vi "Measurement Logic.vi"() -> ()   [LabVIEW 2020, in "IVI Scope Measurement.lvlib"]
uses:
  IVI Scope Measurement.lvlib
  Measurement Configuration.ctl
  Measurement Results.ctl
  <vilib>/MeasurementLink/MeasurementLink Measurement Server/Measure Call Context/Measure Call Context.lvclass
  <vilib>/MeasurementLink/MeasurementLink Measurement Server/Measure Call Context/Reserve Sessions - 1Pin.vi
  IVI Scope Instrument/IVI Scope Instrument.lvlib
  <vilib>/MeasurementLink/MeasurementLink Session Management V1/Session Reservation/Session Reservation.lvclass
panel:
  out "measure call context out":refnum<class "Measure Call Context.lvclass">
  in  "measure call context in":refnum<class "Measure Call Context.lvclass">
  out "measurement results":T1
  in  "measurement configuration":T2={"Pin Name"="", "Time Per Record"=0.0, "Minimum Record Length"=0, "Trigger Level"=0.0, "Vertical Range"=0.0, "Vertical Offset"=10.0, "Probe Attenuation"=1.0, "Vertical Coupling"=1} {"Vertical Coupling" items=["AC", "DC", "GND"]}
  out "error out":errorcluster
  in  "error in":errorcluster
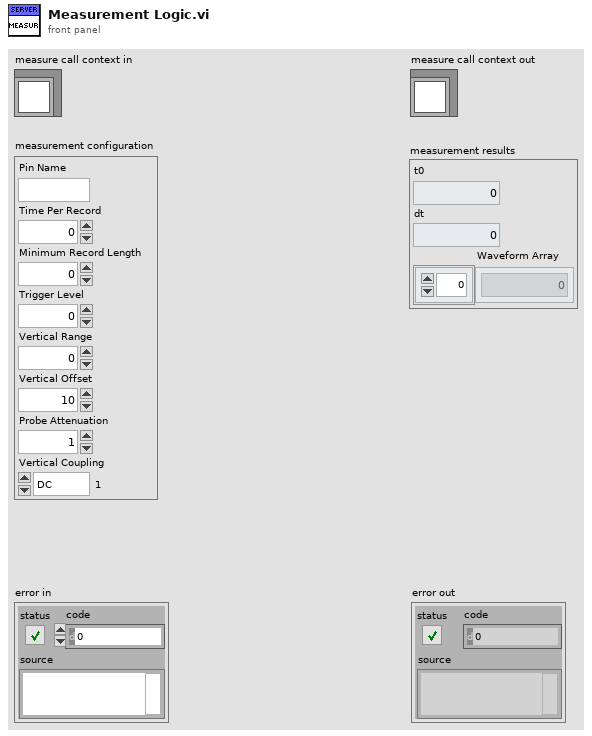
[diagram p1: front panel]
types:
  T1 = typedef "IVI Scope Measurement.lvlib/Measurement Results.ctl" = cluster{"t0":dbl, "dt":dbl, "Waveform Array":dbl[]}
  T2 = typedef "IVI Scope Measurement.lvlib/Measurement Configuration.ctl" = cluster{"Pin Name":string, "Time Per Record":dbl, "Minimum Record Length":i32, "Trigger Level":dbl, "Vertical Range":dbl, "Vertical Offset":dbl, "Probe Attenuation":dbl, "Vertical Coupling":u32}
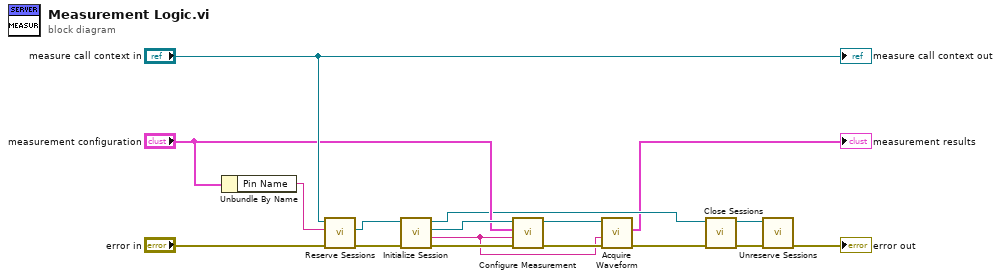
[diagram p0: block diagram]
diagram:
  n1 = Unbundle By Name("measurement configuration") -> ("Pin Name"=w16:string)
  n2 = call-poly <vilib>:"Reserve Sessions.vi"("error in"="error in", "pin or relay name"=w16, "measurement context in"="measure call context in") -> ("error out"=w13:errorcluster, "session reservation out"=w15:refnum<class "Session Reservation.lvclass">)  [unwired: 6 in, 1 out]
  n3 = call "Initialize Session.vi"("error in"=w13, "session reservation in"=w15) -> ("error out"=w12:errorcluster, "channel list"=w1:string, "session"=w11:refnum<k15>, "session reservation out"=w5:refnum<class "Session Reservation.lvclass">)  [unwired: 6 in]
  n4 = call "Configure Measurement.vi"("error in (no error)"=w12, "Channel Name"=w1, "measurement configuration"="measurement configuration", "IVI Refnum in"=w11) -> ("error out"=w9:errorcluster, "IVI Refnum out"=w8:refnum<k15>)  [unwired: 6 in]
  n5 = call "Acquire Waveform.vi"("error in (no error)"=w9, "channel list"=w1, "IVI Refnum in"=w8) -> ("error out"=w4:errorcluster, "Measurement Results"=→"measurement results":T1)  [unwired: 6 in, 1 out]
  n6 = call <vilib>:"Close Sessions.vi"("error in"=w4, "session reservation in"=w5) -> ("error out"=w7:errorcluster, "session reservation out"=w6:refnum<class "Session Reservation.lvclass">)  [unwired: 8 in]
  n7 = call <vilib>:"Unreserve Sessions.vi"("error in"=w7, "session reservation in"=w6) -> ("error out"=→"error out":errorcluster)  [unwired: 9 in]
  "measure call context out" <- "measure call context in"
